vi "SVG Parser.vi"(5 "XML File Path":path, 7 "error in (no error)":errorcluster) -> (0 "Image Size":cluster{"Width":dbl, "Height":dbl}, 1 "rects":T3(array[cluster]), 2 "Funnel":T2(array[cluster]), 3 "Path":T2(array[cluster]), 4 "error out":errorcluster)   [LabVIEW 2013]
doc: "This VI parses an SVG file using LabVIEW's built-in XML parser. It outputs the objects found in an SVG file as well as the canvas width and height."
uses:
  <vilib>/Analysis/Matrix/Datatypes/RealMatrix.ctl
  <vilib>/Analysis/Matrix/NI_Matrix.lvlib
panel:
  out "Order":i32
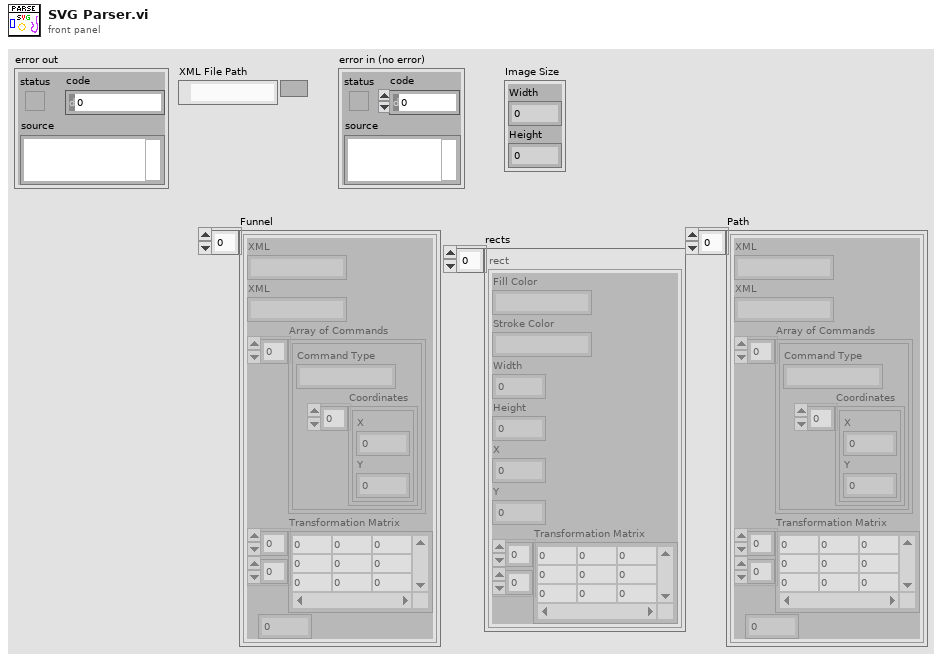
[diagram p1: front panel]
types:
  T1 = typedef "NI_Matrix.lvlib/RealMatrix.ctl" = dbl[][]
  T2 = cluster{"XML":string, "XML":string, "Array of Commands":cluster{"Command Type":string, "Coordinates":cluster{"X":dbl, "Y":dbl}[]}[], "Transformation Matrix":T1, "Order":i32}[]
  T3 = cluster{"Fill Color":string, "Stroke Color":string, "Width":dbl, "Height":dbl, "X":dbl, "Y":dbl, "Transformation Matrix":T1}[]
  T4 = cluster{"XML":string, "XML":string, "Array of Commands":cluster{"Command Type":string, "Coordinates":cluster{"X":dbl, "Y":dbl}[]}[], "Transformation Matrix":T1, i32}[]
  T5 = cluster{"Command Type":string, "Coordinates":cluster{"X":dbl, "Y":dbl}[]}[]
  T6 = cluster{"XML":string, "XML":string, "Array of Commands":cluster{"Command Type":string, "Coordinates":cluster{"X":dbl, "Y":dbl}[]}[], "Transformation Matrix":T1, "Order":i32}
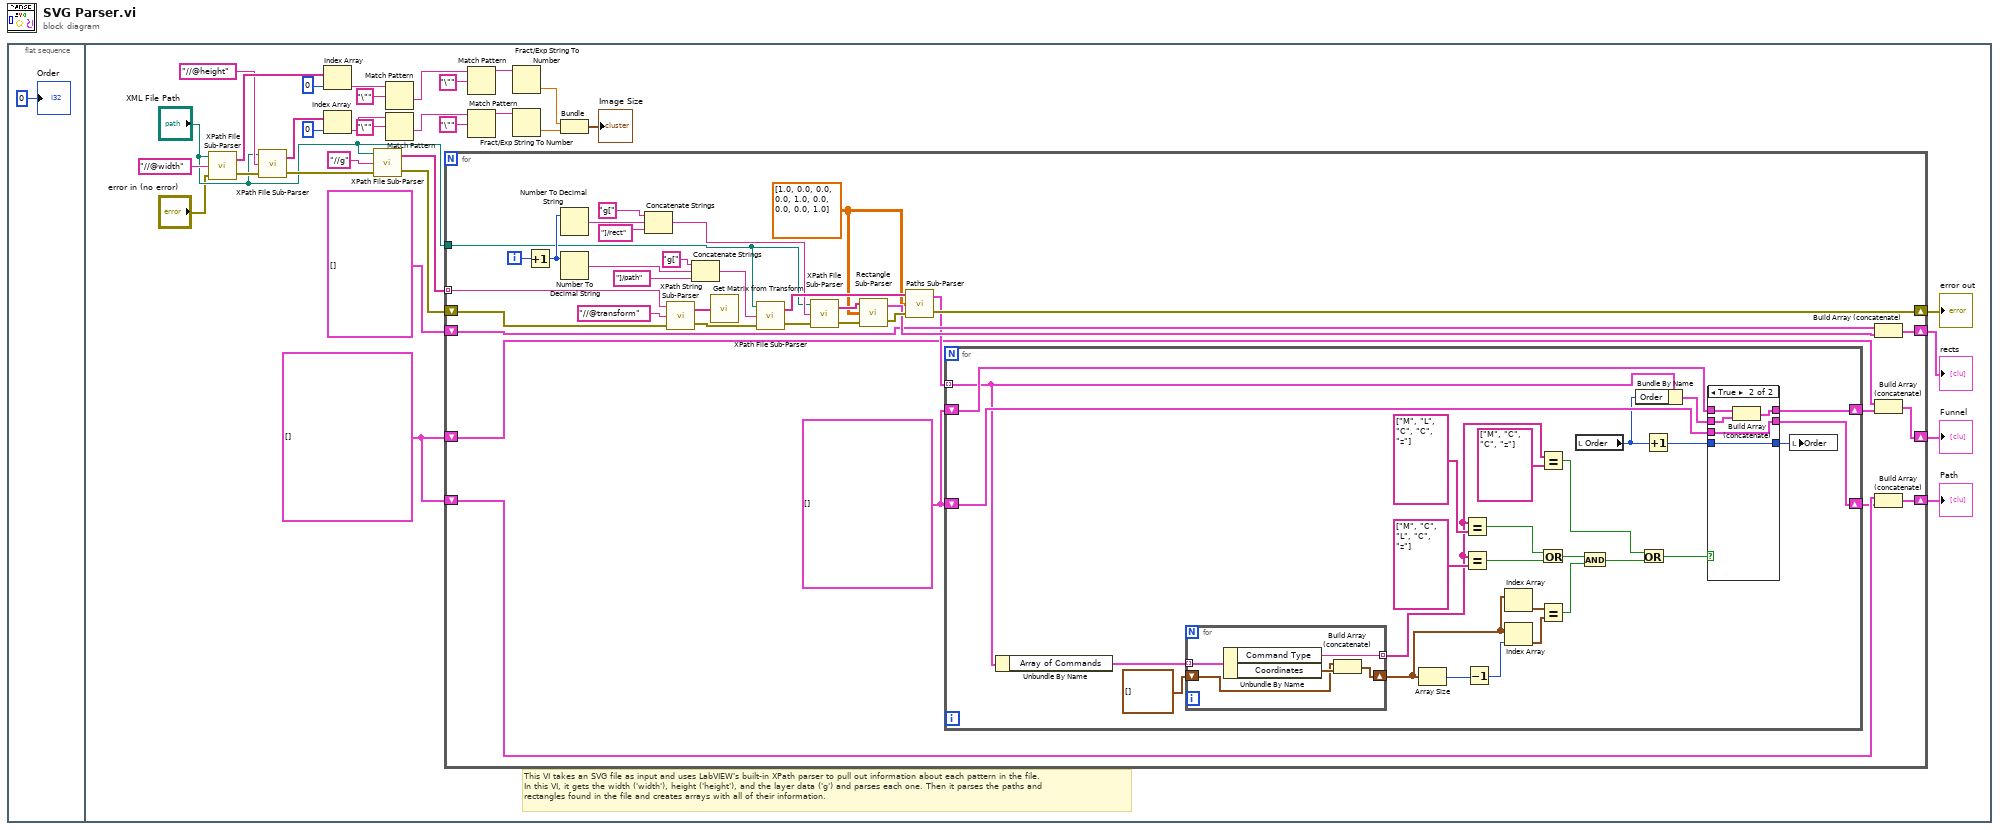
[diagram p0: block diagram]
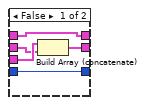
[diagram p2: hidden frame]
diagram:
  n1 = flat-sequence {
    frame #0 {
      "Order" <- 0 ("Order")
    }
    frame #1 {
      w2 = T4 []
      # "This VI takes an SVG file as input and uses LabVIEW's built-in XPath parser to pull out information about each pattern in the file. \nIn this VI, it gets the width ('width'), height ('height'), and the layer data ('g') and parses each one. Then it parses the paths and \nrectangles found in the file and creates arrays with all of their information."
      n2 = call "XPath File Sub-Parser.vi"("error in (no error)"="error in (no error)", "XPath Expression"="//@width" ("XPath expression"), "XML File Path"="XML File Path") -> ("error out"=w27:errorcluster, "Array of Results"=w32:string[])
      n3 = call "XPath File Sub-Parser.vi"("error in (no error)"=w27, "XPath Expression"="//@height" ("XPath expression"), "XML File Path"="XML File Path") -> ("error out"=w15:errorcluster, "Array of Results"=w29:string[])
      n4 = Index Array(array=w32, index=0) -> (element=w22:string)
      n5 = Index Array(array=w29, index=0) -> (element=w17:string)
      n6 = call "XPath File Sub-Parser.vi"("error in (no error)"=w15, "XPath Expression"="//g" ("XPath expression"), "XML File Path"="XML File Path") -> ("error out"=w12:errorcluster, "Array of Results"=w14:string[])
      n7 = Match Pattern(string=w22, regular expression="\"") -> (after substring=w25:string)  [unwired: 1 in, 3 out]
      n8 = Match Pattern(string=w17, regular expression="\"") -> (after substring=w19:string)  [unwired: 1 in, 3 out]
      n9 = for {
        tunnel: w14 -> [w60] mode=indexing
        tunnel: "XML File Path" -> [w44]
        shift-right: [w61] -> w10
        shift-left: w12 -> [w54]
        shift-right: [w56] -> w9
        shift-left: T3 [] -> [w55]
        shift-right: [w40] -> w4
        shift-left: w2 -> [w41]
        shift-right: [w38] -> w3
        shift-left: w2 -> [w37]
        i -> [w46]
        w34 = T1 [[1.0, 0.0, 0.0], [0.0, 1.0, 0.0], [0.0, 0.0, 1.0]] ("Transformation Matrix")
        w35 = T4 []
        n10 = Increment(x=w46) -> (x+1=w45:i32)
        n11 = Number To Decimal String(number=w45) -> (decimal integer string=w48:string)  [unwired: 1 in]
        n12 = Number To Decimal String(number=w45) -> (decimal integer string=w66:string)  [unwired: 1 in]
        n13 = Concatenate Strings("g[" ("string"), w48, "]/rect" ("string")) -> (w47:string)
        n14 = call "XPath String Sub-Parser.vi"("error in (no error)"=w54, "XPath expression"="//@transform", "XML String"=w60) -> ("error out"=w53:errorcluster, "Array of Results"=w58:string[])
        n15 = Concatenate Strings("g[" ("string"), w66, "]/path" ("string")) -> (w67:string)
        n16 = call "Get Matrix from Transform.vi"("Transform Attributes"=w58) -> ()  [unwired: 1 out]
        n17 = call "XPath File Sub-Parser.vi"("error in (no error)"=w53, "XPath Expression"=w67, "XML File Path"=w44) -> ("error out"=w52:errorcluster, "Array of Results"=w51:string[])
        n18 = call "XPath File Sub-Parser.vi"("error in (no error)"=w52, "XPath Expression"=w47, "XML File Path"=w44) -> ("error out"=w43:errorcluster, "Array of Results"=w62:string[])
        n19 = call "Rectangle Sub-Parser.vi"("error in (no error)"=w43, "Transformation Matrix"=w34, "Array of Nodes"=w62) -> ("error out"=w63:errorcluster, "rects"=w57:T3)
        n20 = call "Paths Sub-Parser.vi"("error in (no error)"=w63, "Transformation Matrix"=w34, "Array of Nodes"=w51) -> ("error out"=w61:errorcluster, "Path"=w42:T2)
        n21 = for {
          tunnel: w42 -> [w88] mode=indexing
          shift-right: [w92] -> w36
          shift-left: w35 -> [w91]
          shift-right: [w90] -> w39
          shift-left: w35 -> [w89]
          n22 = Unbundle By Name(w88) -> ("Array of Commands"=w93:T5)
          n23 = for {
            tunnel: w93 -> [w109] mode=indexing
            tunnel: [w108] -> w75 mode=indexing
            shift-right: [w106] -> w83
            shift-left: cluster{"X":dbl, "Y":dbl}[] [] -> [w105]
            n24 = Unbundle By Name(w109) -> ("Command Type"=w108:string, "Coordinates"=w107:cluster{"X":dbl, "Y":dbl}[])
            n25 = Build Array (concatenate)(w105, w107) -> (w106:cluster{"X":dbl, "Y":dbl}[])
          }
          n26 = Array Size(array=w83) -> (size(s)=w78:i32)
          n27 = Equal?(x=w75, y=string[] ["M", "L", "C", "C", "z"]) -> (x = y?=w69:bool)
          n28 = Equal?(x=w75, y=string[] ["M", "C", "L", "C", "z"]) -> (x = y?=w68:bool)
          n29 = Decrement(x=w78) -> (x-1=w77:i32)
          n30 = Index Array(array=w83) -> (element=w82:cluster{"X":dbl, "Y":dbl})  [unwired: 1 in]
          n31 = Index Array(array=w83, index=w77) -> (element=w81:cluster{"X":dbl, "Y":dbl})
          n32 = Equal?(x=w75, y=string[] ["M", "C", "C", "z"]) -> (x = y?=w70:bool)
          n33 = Or(x=w69, y=w68) -> (x .or. y?=w74:bool)
          n34 = Equal?(x=w82, y=w81) -> (x = y?=w80:bool)
          n35 = local read "Order"() -> (w73:i32)
          n36 = And(x=w74, y=w80) -> (x .and. y?=w79:bool)
          n37 = Bundle By Name(cluster=w88, "Order"=w73) -> (w87:T6)
          n38 = Or(x=w70, y=w79) -> (x .or. y?=w85:bool)
          n39 = Increment(x=w73) -> (x+1=w72:i32)
          n40 = case shown="True" w85 {
            tunnel: w87 -> [w97 w102]
            tunnel: [w99 w101] -> w92
            tunnel: w91 -> [w98 w101]
            tunnel: [w96 w104] -> w90
            tunnel: w89 -> [w96 w103]
            tunnel: w72 -> [w95 w100]
            tunnel: [w95 w100] -> w71
            frame False {
              n41 = Build Array (concatenate)(w98, w97) -> (w99:T2)
            }
            frame True {
              n42 = Build Array (concatenate)(w103, w102) -> (w104:T2)
            }
          }
          n43 = local write "Order"(w71) -> ()
        }
        n44 = Build Array (concatenate)(w55, w57) -> (w56:T3)
        n45 = Build Array (concatenate)(w37, w39) -> (w38:T4)
        n46 = Build Array (concatenate)(w41, w36) -> (w40:T4)
      }
      "error out" <- w10
      "rects" <- w9
      "Path" <- w4
      "Funnel" <- w3
      n47 = Match Pattern(string=w25, regular expression="\"") -> (before substring=w23:string)  [unwired: 1 in, 3 out]
      n48 = Match Pattern(string=w19, regular expression="\"") -> (before substring=w21:string)  [unwired: 1 in, 3 out]
      n49 = Fract/Exp String To Number(string=w23) -> (number=w6:dbl)  [unwired: 3 in, 1 out]
      n50 = Fract/Exp String To Number(string=w21) -> (number=w7:dbl)  [unwired: 3 in, 1 out]
      n51 = Bundle(w6, w7) -> (→"Image Size":cluster{dbl, dbl})  [unwired: 1 in]
    }
  }
